vi "Day 02 (Part Two).vi"() -> ()   [LabVIEW 2021]
panel:
  out "result":i32
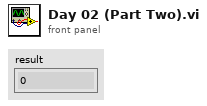
[diagram p1: front panel]
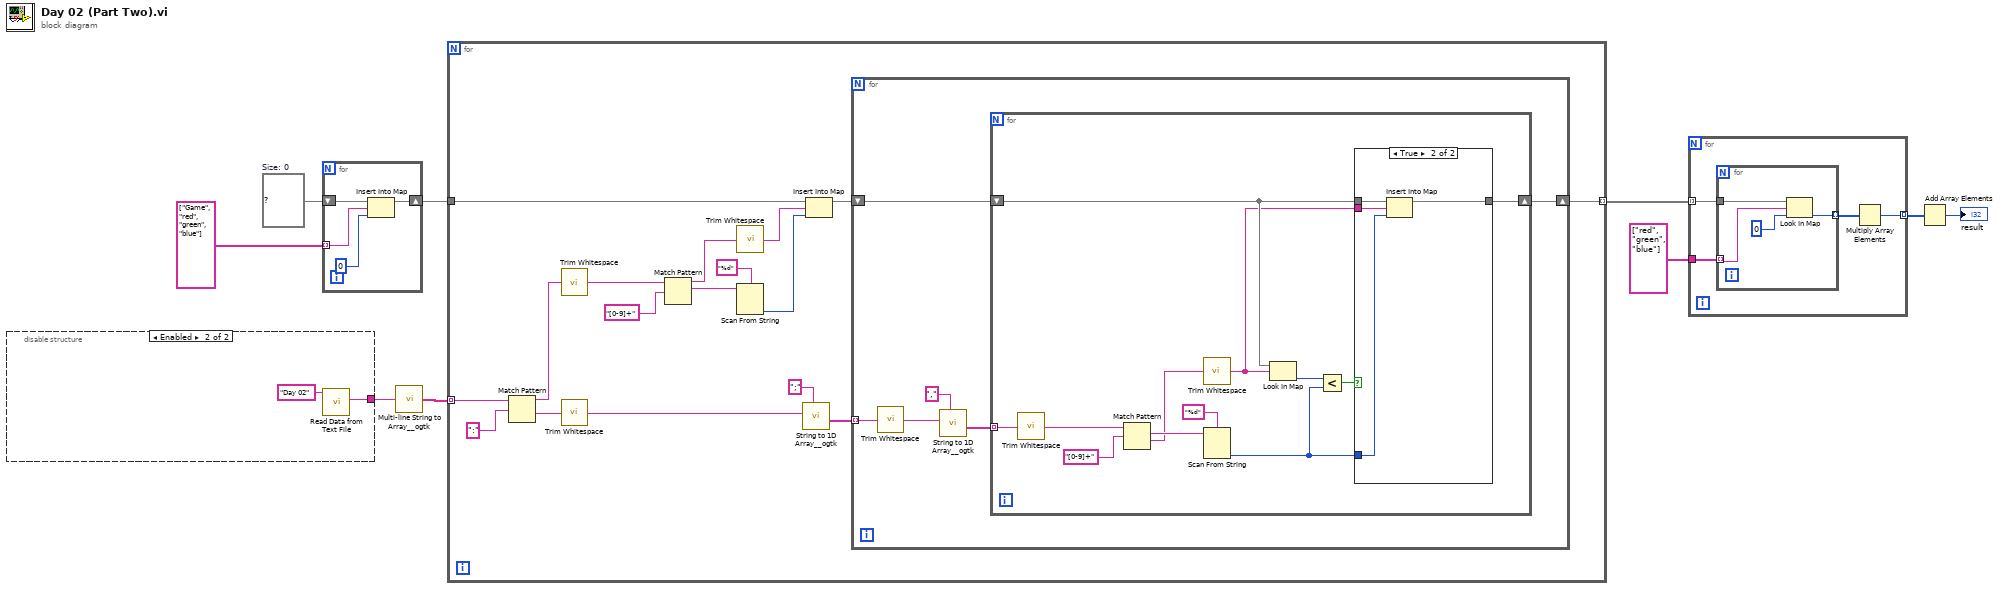
[diagram p0: block diagram]
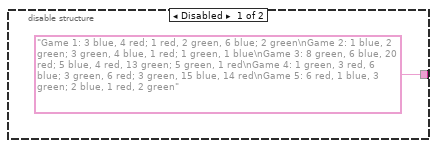
[diagram p3: hidden frame]
diagram:
  w6 = map{string, i32} {}  # Size: 0
  n1 = disable-structure shown="Enabled" {
    disable-tunnel: ["Game 1: 3 blue, 4 red; 1 red, 2 green, 6 blue; 2 green\nGame 2: 1 blue, 2 green; 3 green, 4 blue, 1 red; 1 green, 1 blue\nGame 3: 8 green, 6 blue, 20 red; 5 blue, 4 red, 13 green; 5 green, 1 red\nGame 4: 1 green, 3 red, 6 blue; 3 green, 6 red; 3 green, 15 blue, 14 red\nGame 5: 6 red, 1 blue, 3 green; 2 blue, 1 red, 2 green" w12] -> w9
    frame Disabled {
    }
    frame Enabled {
      n2 = call "Read Data from Text File.vi"("Subfolder"="Day 02") -> ("data"=w12:string)  [unwired: 10 in]
    }
  }
  n3 = for {
    tunnel: string[] ["Game", "red", "green", "blue"] -> [w16] mode=indexing
    shift-right: [w13] -> w5
    shift-left: w6 -> [w14]
    n4 = Insert Into Map(map in=w14, key=w16, value=0) -> (map out=w13:map{string, i32})  [unwired: 2 out]
  }
  n5 = call <userlib>:"Multi-line String to Array__ogtk.vi"("string"=w9) -> ("lines"=w8:string[])
  n6 = for {
    tunnel: w8 -> [w33] mode=indexing
    tunnel: w5 -> [w26]
    tunnel: [w17] -> w4 mode=indexing
    n7 = Match Pattern(string=w33, regular expression=":") -> (before substring=w31:string, after substring=w30:string)  [unwired: 1 in, 2 out]
    n8 = call <vilib>:"Trim Whitespace.vi"("string"=w31) -> ("trimmed string"=w24:string)  [unwired: 1 in]
    n9 = call <vilib>:"Trim Whitespace.vi"("string"=w30) -> ("trimmed string"=w29:string)  [unwired: 1 in]
    n10 = Match Pattern(string=w24, regular expression="[0-9]+") -> (before substring=w22:string, match substring=w21:string)  [unwired: 1 in, 2 out]
    n11 = call <vilib>:"Trim Whitespace.vi"("string"=w22) -> ("trimmed string"=w19:string)  [unwired: 1 in]
    n12 = Scan From String(format string="%d", input string=w21) -> (output 1=w20:i32)  [unwired: 3 in, 3 out]
    n13 = call <userlib>:"String to 1D Array__ogtk.vi"("delimiter (Tab)"=";", "string"=w29) -> ("Array of Strings"=w27:string[])  [unwired: 9 in]
    n14 = Insert Into Map(map in=w26, key=w19, value=w20) -> (map out=w18:map{string, i32})  [unwired: 2 out]
    n15 = for {
      tunnel: w27 -> [w39] mode=indexing
      shift-right: [w34] -> w17
      shift-left: w18 -> [w35]
      n16 = call <vilib>:"Trim Whitespace.vi"("string"=w39) -> ("trimmed string"=w37:string)  [unwired: 1 in]
      n17 = call <userlib>:"String to 1D Array__ogtk.vi"("delimiter (Tab)"=",", "string"=w37) -> ("Array of Strings"=w36:string[])  [unwired: 9 in]
      n18 = for {
        tunnel: w36 -> [w51] mode=indexing
        shift-right: [w40] -> w34
        shift-left: w35 -> [w43]
        n19 = call <vilib>:"Trim Whitespace.vi"("string"=w51) -> ("trimmed string"=w50:string)  [unwired: 1 in]
        n20 = Match Pattern(string=w50, regular expression="[0-9]+") -> (match substring=w48:string, after substring=w46:string)  [unwired: 1 in, 2 out]
        n21 = call <vilib>:"Trim Whitespace.vi"("string"=w46) -> ("trimmed string"=w42:string)  [unwired: 1 in]
        n22 = Scan From String(format string="%d", input string=w48) -> (output 1=w41:i32)  [unwired: 3 in, 3 out]
        n23 = Look In Map(map=w43, key=w42) -> (value=w45:i32)  [unwired: 1 in, 1 out]
        n24 = Less?(x=w45, y=w41) -> (x < y?=w44:bool)
        n25 = case shown="True" w44 {
          tunnel: w43 -> [w52 w56]
          tunnel: w42 -> [_ w55]
          tunnel: w41 -> [_ w54]
          tunnel: [w52 w53] -> w40
          frame False {
          }
          frame True {
            n26 = Insert Into Map(map in=w56, key=w55, value=w54) -> (map out=w53:map{string, i32})  [unwired: 2 out]
          }
        }
      }
    }
  }
  n27 = for {
    tunnel: w4 -> [w59] mode=indexing
    tunnel: string[] ["red", "green", "blue"] -> [w60]
    tunnel: [w57] -> w2 mode=indexing
    n28 = for {
      tunnel: w59 -> [w64]
      tunnel: w60 -> [w63] mode=indexing
      tunnel: [w61] -> w58 mode=indexing
      n29 = Look In Map(map=w64, key=w63, default value=0) -> (value=w61:i32)  [unwired: 1 out]
    }
    n30 = Multiply Array Elements(1:w58) -> (0:w57:i32)
  }
  n31 = Add Array Elements(numeric array=w2) -> (sum=→"result":i32)
